vi "Test File Sink Default Logger.vi"(11 "Test Case In":refnum<class "File Sink.lvclass">) -> (0 "error out":errorcluster, 3 "Test Case Out":refnum<class "File Sink.lvclass">)   [LabVIEW 2020, in "File Sink.lvclass"]
uses:
  File Sink.lvclass
  C:/Program Files (x86)/National Instruments/LabVIEW 2020/vi.lib/Astemes/LUnit/Test Case.lvclass
  Source/Type Defs/Debug Level.ctl
  <vilib>/Astemes/LUnit/Test Case.lvclass/Test Case.ctl
  e94ff1bf-c1b1-42c1-a6e3-1538fdc900a3.vi
  4993e8ee-a06a-463a-9684-69129f64d5ce.vi
  ebeb964f-1c40-45c4-b7ad-328f89dac856.vi
  <vilib>/Astemes/LUnit/Core/LUnit Test Case/Private/Append Pass Result.vi
  <vilib>/Astemes/LUnit/Core/LUnit Test Case/Private/Append Fail Result.vi
  e94ff1bf-c1b1-42c1-a6e3-1538fdc900a3.vi/9c5d11cd-9439-4240-a1ee-d9baace9c924.vi
  4993e8ee-a06a-463a-9684-69129f64d5ce.vi/9c5d11cd-9439-4240-a1ee-d9baace9c924.vi
  ebeb964f-1c40-45c4-b7ad-328f89dac856.vi/9c5d11cd-9439-4240-a1ee-d9baace9c924.vi
  <vilib>/Astemes/LUnit/Core/LUnit Test Case/Private/Run In UI.vi
  <vilib>/Utility/error.llb/Clear Errors.vi
  Source/Sinks/File Sink/File Sink.lvclass
  C:/Users/hughe_cx/Documents/05_repos/LVLog/Source/Sinks/Sink/Sink.lvclass
  <vilib>/Astemes/LUnit/Test Case.lvclass
  Source/LV Log.lvlib
  Source/Logger/Logger.lvclass
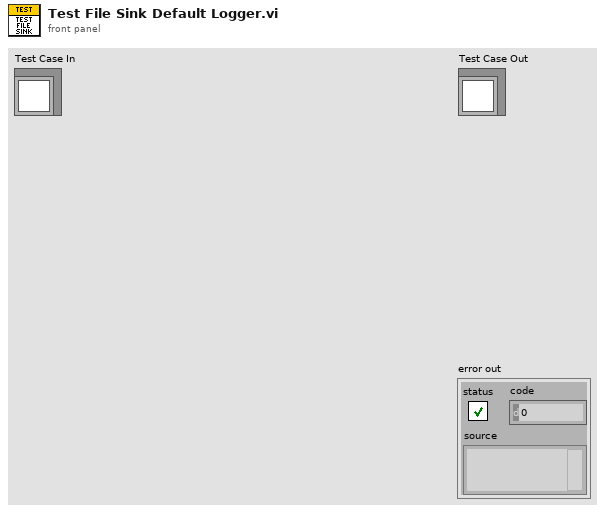
[diagram p1: front panel]
types:
  T1 = typedef "LV Log.lvlib/Debug Level.ctl" = enum16{"DEFAULT", "DEBUG", "INFO", "WARN", "ERROR", "FATAL"}
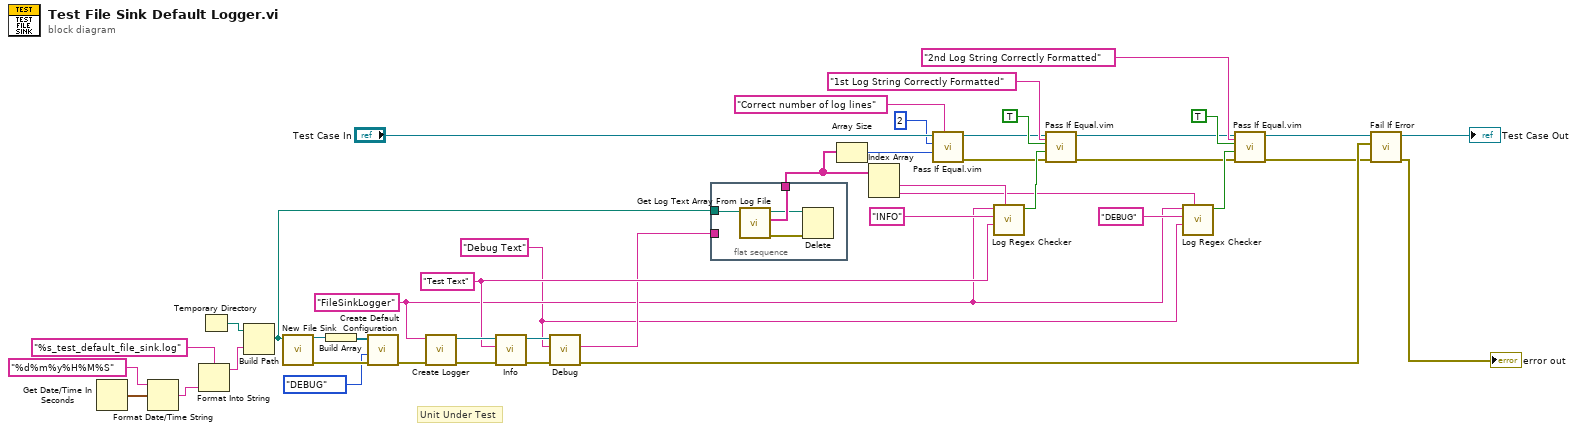
[diagram p0: block diagram]
diagram:
  w14 = "Debug Text" ("Log Text")
  w26 = "Test Text" ("Log Text")
  w15 = "FileSinkLogger" ("Name")
  # "Unit Under Test"
  n1 = Get Date/Time In Seconds() -> (seconds since 1Jan1904=w35:timestamp)
  n2 = Format Date/Time String(time format string (%c)="%d%m%y%H%M%S", seconds (now)=w35) -> (date/time string=w33:string)  [unwired: 1 in]
  n3 = Format Into String(format string="%s_test_default_file_sink.log", w33) -> (resulting string=w36:string)  [unwired: 2 in, 1 out]
  n4 = Temporary Directory() -> (w38:path)
  n5 = Build Path(base path=w38, name or relative path=w36) -> (appended path=w29:path)
  n6 = call "New File Sink.vi"("File Path"=w29) -> ("error out"=w41:errorcluster, "File Sink out"=w39:refnum<class "File Sink.lvclass">)  [unwired: 9 in]
  n7 = Build Array(w39) -> (w40:refnum<class "File Sink.lvclass">[])
  n8 = call "Create Default Configuration.vi"("Sinks"=w40, "Debug Level in"=Debug_Level."DEBUG", "error in (no error)"=w41) -> ("error out"=w42:errorcluster)  [unwired: 7 in]
  n9 = call "Create Logger.vi"("error in (no error)"=w42, "Name"=w15) -> ("error out"=w31:errorcluster, "Logger out"=w30:refnum<class "Logger.lvclass">)  [unwired: 8 in]
  n10 = call "Info.vi"("error in (no error)"=w31, "Log Text"=w26, "Logger in"=w30) -> ("error out"=w25:errorcluster, "Logger out"=w24:refnum<class "Logger.lvclass">)  [unwired: 6 in, 1 out]
  n11 = call "Debug.vi"("error in (no error)"=w25, "Log Text"=w14, "Logger in"=w24) -> ("error out"=w23:errorcluster, "Log Output"=w22:string)  [unwired: 6 in, 1 out]
  n12 = flat-sequence {
    tunnel: w29 -> [w48]
    tunnel: w22 -> [_]
    tunnel: [w47] -> w7
    frame #0 {
      n13 = call "Get Log Text Array From Log File.vi"("Log File Path in"=w48) -> ("error out"=w46:errorcluster, "Log Text Array"=w47:string[], "Log File Path out"=w45:path)  [unwired: 8 in]
      n14 = Delete(path (use dialog)=w45, error in=w46) -> ()  [unwired: 3 in, 3 out]
    }
  }
  n15 = Array Size(array=w7) -> (size(s)=w6:i32)
  n16 = Index Array(array=w7) -> (element #1=w13:string, element #2=w12:string)  [unwired: 2 in]
  n17 = call "Pass If Equal.vim"("Description"="Correct number of log lines", "Actual"=w6, "Expected"=2, "LUnit Test Case In"="Test Case In") -> ("error out"=w1:errorcluster, "LUnit Test Case Out"=w9:refnum<class "File Sink.lvclass">)  [unwired: 6 in]
  n18 = call "Log Regex Checker.vi"("Log String"=w13, "Expected Log Text (Any)"=w26, "Expected Log Level (Any)"="INFO", "Expected Logger Name (Any)"=w15) -> ("Math Found"=w20:bool)  [unwired: 5 in, 2 out]
  n19 = call "Pass If Equal.vim"("Description"="1st Log String Correctly Formatted", "error in (no error)"=w1, "Actual"=w20, "Expected"=TRUE, "LUnit Test Case In"=w9) -> ("error out"=w2:errorcluster, "LUnit Test Case Out"=w11:refnum<class "File Sink.lvclass">)  [unwired: 5 in]
  n20 = call "Log Regex Checker.vi"("Log String"=w12, "Expected Log Text (Any)"=w14, "Expected Log Level (Any)"="DEBUG", "Expected Logger Name (Any)"=w15) -> ("Math Found"=w19:bool)  [unwired: 5 in, 2 out]
  n21 = call "Pass If Equal.vim"("Description"="2nd Log String Correctly Formatted", "error in (no error)"=w2, "Actual"=w19, "Expected"=TRUE, "LUnit Test Case In"=w11) -> ("error out"=w3:errorcluster, "LUnit Test Case Out"=w10:refnum<class "File Sink.lvclass">)  [unwired: 5 in]
  n22 = call <vilib>:"Fail If Error.vi"("error in (no error)"=w3, "Assert error"=w23, "LUnit Test Case In"=w10) -> ("error out"=→"error out":errorcluster, "LUnit Test Case Out"=→"Test Case Out":refnum<class "File Sink.lvclass">)  [unwired: 7 in]
